vi "weather array.vi"(9 "Array":i8[](array[numeric]), 10 "数组":T1(array[cluster])) -> (2 "Array 2":i8[](array[numeric]))   [LabVIEW 2018]
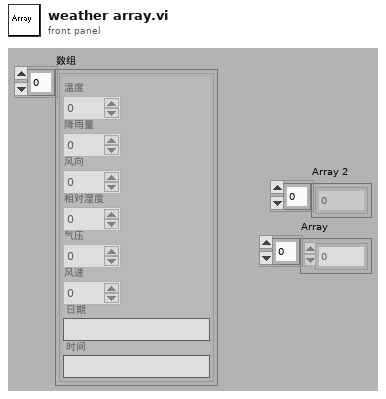
[diagram p1: front panel]
types:
  T1 = cluster{"温度":dbl, "降雨量":dbl, "风向":dbl, "相对湿度":dbl, "气压":dbl, "风速":dbl, "日期":string, "时间":string}[]
  T2 = cluster{"温度":dbl, "降雨量":dbl, "风向":dbl, "相对湿度":dbl, "气压":dbl, "风速":dbl, "日期":string, "时间":string}
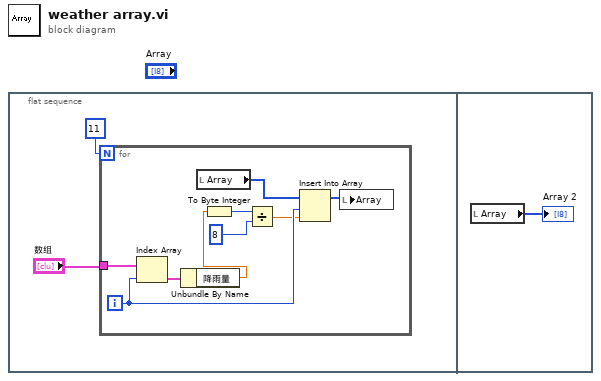
[diagram p0: block diagram]
diagram:
  n1 = flat-sequence {
    frame #0 {
      n2 = for {
        N: 11 -> [_]
        tunnel: "数组" -> [w4]
        i -> [w6]
        n3 = Index Array(array=w4, index=w6) -> (element=w11:T2)
        n4 = Unbundle By Name(w11) -> ("降雨量"=w10:dbl)
        n5 = local read "Array"() -> (w3:i8[])
        n6 = To Byte Integer(number=w10) -> (8bit integer=w9:i8)
        n7 = Divide(x=w9, y=i8 8) -> (x/y=w5:dbl)
        n8 = Insert Into Array(array=w3, index=w6, new element=w5) -> (w7:i8[])
        n9 = local write "Array"(w7) -> ()
      }
    }
    frame #1 {
      n10 = local read "Array"() -> (→"Array 2":i8[])
    }
  }
